vi "LV SCISDK Read Custom Packet Multiple Data.vi"(0 "Path":string, 1 "buffer size":u32, 2 "handle":u64, 3 "error in (no error)":errorcluster) -> (7 "function return":i32, 8 "buffer out":T1, 9 "handle out":u64, 10 "error out":errorcluster)   [LabVIEW 2021, in "SciSDK_Labview.lvlib"]
doc: "SCISDKLABVIEW_DLL_API int LV_SCISDK_ReadData(char* Path, LV_OSCILLOSCOPE_DECODED_BUFFER* buffer, void* handle);"
uses:
  SciSDK_Labview.lvlib
panel:
  in  "buffer":T2
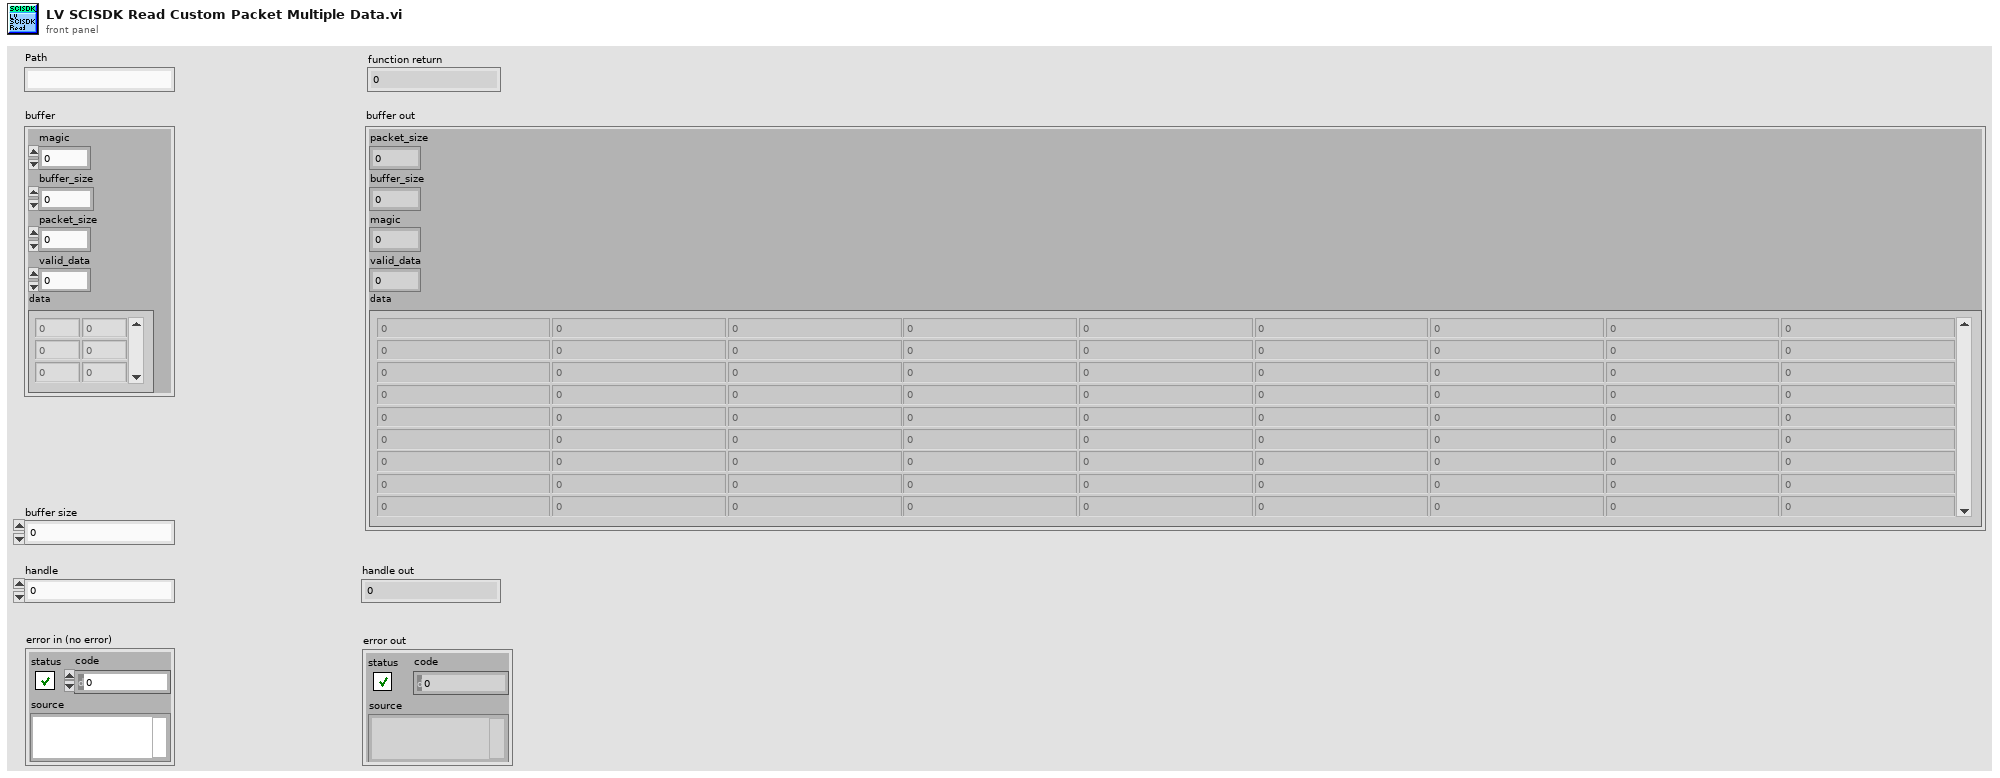
[diagram p1: front panel]
types:
  T1 = cluster{"packet_size":u32, "buffer_size":u32, "magic":u32, "valid_data":dbl, "data":u32[][]}
  T2 = cluster{"magic":u32, "buffer_size":u32, "packet_size":u32, "valid_data":u32, "data":u32[][]}
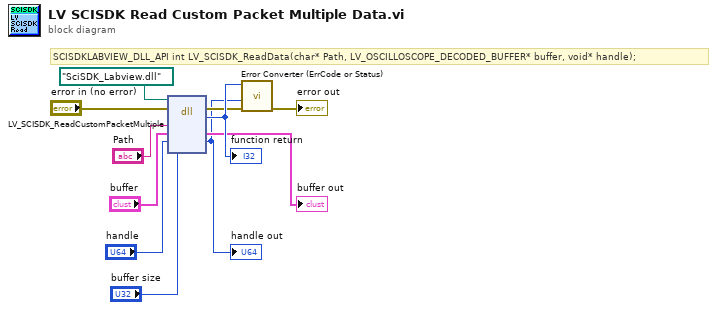
[diagram p0: block diagram]
diagram:
  # "SCISDKLABVIEW_DLL_API int LV_SCISDK_ReadData(char* Path, LV_OSCILLOSCOPE_DECODED_BUFFER* buffer, void* handle);"
  n1 = dll-call lib="C:/git/scisdk/SciSDK_VC++/x64/Debug/SciSDK_Labview.dll" fn="LV_SCISDK_ReadCustomPacketMultiple"(path in=path "SciSDK_Labview.dll", error in="error in (no error)", "Path"="Path", "buffer"="buffer", "handle"="handle", "buffer_size"="buffer size") -> (error out=w7:errorcluster, "return type"=w11:i32, "buffer"=→"buffer out":T2, "handle"=w1:u64)  [unwired: 3 in, 1 out]
  "function return" <- w11
  "handle out" <- w1
  n2 = call "Error Converter (ErrCode or Status).vi"("error in (no error)"=w7, "handle"=w1, "error code"=w11) -> ("error out"=→"error out":errorcluster)  [unwired: 8 in]
